vi "ProjectConnect.vi"(8 "error in (no error)":errorcluster, 11 "Project Ref in":T1) -> (0 "error out":errorcluster, 3 "Project Ref out":T1)   [LabVIEW 2015, in "MiscHelperVIs.lvlib"]
uses:
  MiscHelperVIs.lvlib
  <vilib>/NI Veristand/Execution/Project/Project Ref.ctl
  NationalInstruments.VeriStand.ClientAPI
  <vilib>/NI Veristand/Execution/Project/NI_VS Project ExecutionAPI.lvlib
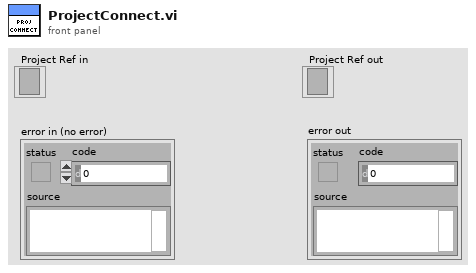
[diagram p1: front panel]
types:
  T1 = typedef "NI_VS Project ExecutionAPI.lvlib/Project Ref.ctl" = refnum<k24>
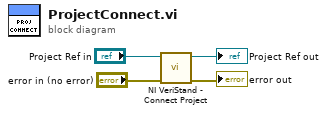
[diagram p0: block diagram]
diagram:
  n1 = call <vilib>:"NI VeriStand - Connect Project.vi"("error in (no error)"="error in (no error)", "Project Ref in"="Project Ref in") -> ("error out"=→"error out":errorcluster, "Project Ref out"=→"Project Ref out":T1)  [unwired: 8 in]
